vi "NI9401_test.vi"() -> ()   [LabVIEW 2014]
uses:
  <vilib>/rvi/Emulation/niFpgaGetClockAttributes.vi
  <vilib>/rvi/Emulation/niFpgaSctlEmulationGetInTimedLoop.vi
  <vilib>/rvi/Emulation/niFpgaEmulationReportErrorSimple.vi
  <vilib>/rvi/eio/common/nirviEmuTemplateMethod_errors.vi
  <vilib>/rvi/Emulation/niFpgaCriticalErrorInLSC.vi
  <vilib>/eio/EIONode/EIONode.xnode
panel:
  in  "Mod8/AO14":fxp<+/-,20,5>
  out "Mod7/DIO7":bool
  out "Mod7/DIO5":bool
  out "Mod7/DIO6":bool
  out "Mod7/DIO4":bool
  out "Mod7/DIO3":bool
  out "Mod7/DIO2":bool
  out "Mod7/DIO1":bool
  out "Mod7/DIO0":bool
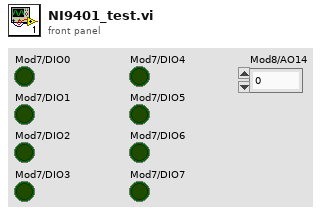
[diagram p1: front panel]
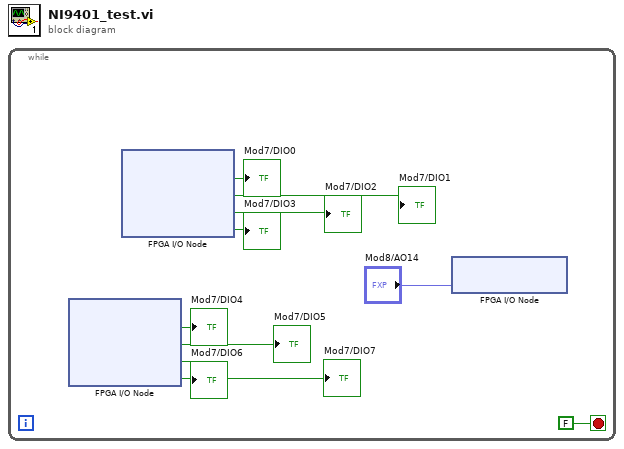
[diagram p0: block diagram]
diagram:
  n1 = while {
    stop <- FALSE stop-if-true
    n2 = xnode "FPGA I/O Node"() -> ("Mod7/DIO4"=→"Mod7/DIO4":bool, "Mod7/DIO5"=→"Mod7/DIO5":bool, "Mod7/DIO6"=→"Mod7/DIO6":bool, "Mod7/DIO7"=→"Mod7/DIO7":bool)  [unwired: 4 in, 4 out]
    n3 = xnode "FPGA I/O Node"() -> ("Mod7/DIO0"=→"Mod7/DIO0":bool, "Mod7/DIO1"=→"Mod7/DIO1":bool, "Mod7/DIO2"=→"Mod7/DIO2":bool, "Mod7/DIO3"=→"Mod7/DIO3":bool)  [unwired: 4 in, 4 out]
    n4 = xnode "FPGA I/O Node"("Mod8/AO14"="Mod8/AO14") -> ()  [unwired: 1 in, 1 out]
  }
